vi "Mirror-TargetConverter.vi"(1 "output unit (target only)":u16(ring) items=["mm", "um"], 8 "axis":u16(ring) items=["X", "Z"], 9 "input units":u16(ring) items=["mm", "um"], 10 "Conversion":u16(ring) items=["t2m", "m2t"], 11 "input distance":dbl) -> (3 "output distance":dbl)   [LabVIEW 2024]
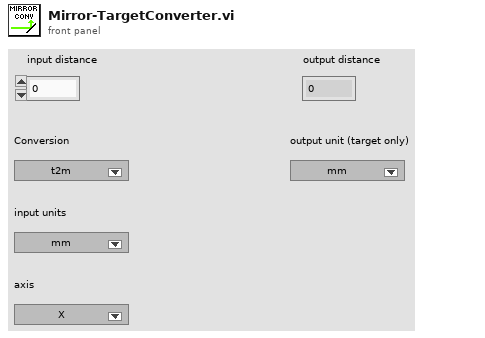
[diagram p1: front panel]
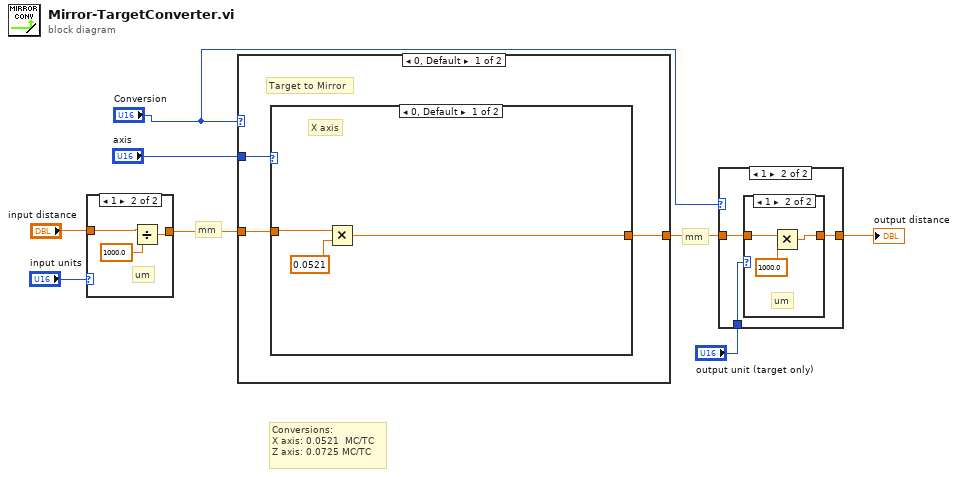
[diagram p0: block diagram]
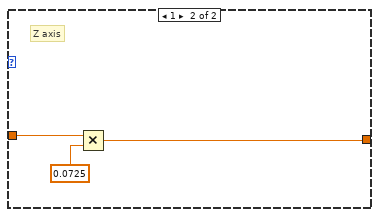
[diagram p5: hidden frame]
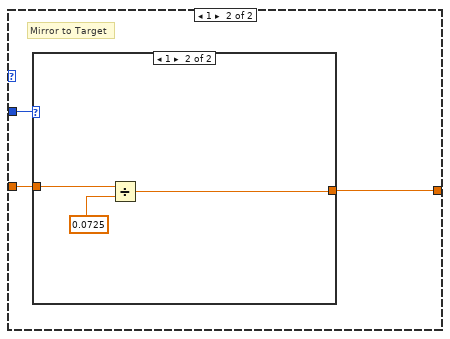
[diagram p6: hidden frame]
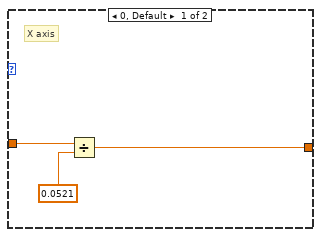
[diagram p7: hidden frame]
diagram:
  # "mm"
  # "Conversions:\nX axis: 0.0521  MC/TC\nZ axis: 0.0725 MC/TC"
  # "mm"
  n1 = case shown="1" "input units" {
    tunnel: [w9 w12] -> w6
    tunnel: "input distance" -> [w9 w11]
    frame 0, Default {
      # "mm"
    }
    frame 1 {
      # "um"
      n2 = Divide(x=w11, y=1000.0) -> (x/y=w12:dbl)
    }
  }
  n3 = case shown="0, Default" "Conversion" {
    tunnel: "axis" -> [w15 w24]
    tunnel: w6 -> [w14 w23]
    tunnel: [w13 w22] -> w3
    frame 0, Default {
      # "Target to Mirror"
      n4 = case shown="0, Default" w15 {
        tunnel: w14 -> [w18 w21]
        tunnel: [w17 w20] -> w13
        frame 0, Default {
          # "X axis"
          n5 = Multiply(x=w18, y=0.0521) -> (x*y=w17:dbl)
        }
        frame 1 {
          # "Z axis"
          n6 = Multiply(x=w21, y=0.0725) -> (x*y=w20:dbl)
        }
      }
    }
    frame 1 {
      # "Mirror to Target"
      n7 = case shown="1" w24 {
        tunnel: w23 -> [w27 w30]
        tunnel: [w25 w29] -> w22
        frame 0, Default {
          # "X axis"
          n8 = Divide(x=w27, y=0.0521) -> (x/y=w25:dbl)
        }
        frame 1 {
          n9 = Divide(x=w30, y=0.0725) -> (x/y=w29:dbl)
        }
      }
    }
  }
  n10 = case shown="1" "Conversion" {
    tunnel: w3 -> [w31 w33]
    tunnel: [w31 w32] -> w2
    tunnel: "output unit (target only)" -> [_ w34]
    frame 0, Default {
    }
    frame 1 {
      n11 = case shown="1" w34 {
        tunnel: w33 -> [w35 w37]
        tunnel: [w35 w38] -> w32
        frame 0, Default {
          # "mm"
        }
        frame 1 {
          # "um"
          n12 = Multiply(x=w37, y=1000.0) -> (x*y=w38:dbl)
        }
      }
    }
  }
  "output distance" <- w2
